vi "Facade.vi"(0 "Data In":T4, 2 "Display State In":T2, 3 "Container State":T3) -> (6 "Data Out":T4, 7 "Display State Out":T2, 8 "Action":T1)   [LabVIEW 2020, in "TTL XCtrl.xctl"]
uses:
  TTL XCtrl.xctl
  Data.vi
  TTL VIs/Control Classes/Base Class/TTLController.lvclass
  <vilib>/_xctls/Container State.ctl
  State.vi
  TTL VIs/Device Classes/Base Class/TTLControlledDevice.lvclass
  D:/Development/epl-vi-lib/Koop/KObject Class/KObject.lvclass
  <vilib>/_xctls/Action.ctl
  TTL VIs/Typedefs/TTLController XControl/TTLController.xctl
  TTL VIs/Control Classes/TTLWaterController/TTLWaterController.lvclass
  D:/Development/epl-tosca/LV Source/TTL VIs/Control Classes/Base Class/TTLController.lvclass
  TTL VIs/Control Classes/Base Class/TTLController.lvclass/TTLController.ctl
  TTL VIs/Device Classes/Base Class/TTLControlledDevice.lvclass/TTLControlledDevice.ctl
  TTL VIs/Control Classes/TCPController/TCPController.lvclass
  TTL VIs/Control Classes/Base Class/Read Name.vi
  TTL VIs/Device Classes/Base Class/Read Name.vi
  TTL VIs/Control Classes/Base Class/Write Name.vi
  <vilib>/_xctls/XControlSupport.lvlib
  epl-vi-lib/Koop/KObject Class/KObject.lvclass
panel:
  in  "TTL1":refnum<class "TTLController.lvclass">(xcontrol)
  in  "TTL2":refnum<class "TTLController.lvclass">(xcontrol)
  in  "TTL3":refnum<class "TTLController.lvclass">(xcontrol)
  in  "TTL4":refnum<class "TTLController.lvclass">(xcontrol)
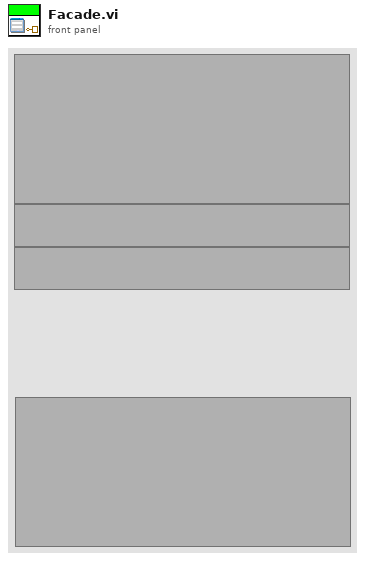
[diagram p1: front panel]
types:
  T1 = typedef "XControlSupport.lvlib/Action.ctl" = cluster{"Data Changed?":bool, "State Changed?":bool, "Action Name":string}
  T2 = typedef "TTL XCtrl.xctl/State.vi" = cluster{"Devices":refnum<class "TTLControlledDevice.lvclass">[], "action":string}
  T3 = typedef "XControlSupport.lvlib/Container State.ctl" = cluster{"Indicator?":bool, "Run Mode?":bool, " Refnum":refnum<vi>}
  T4 = typedef "TTL XCtrl.xctl/Data.vi" = refnum<class "TTLController.lvclass">[]
  T5 = enum16{"Always On", "Always Off", "Off While Running"}
  T6 = typedef "LVRectTypeDef.ctl" = cluster{"Left":i16, "Top":i16, "Right":i16, "Bottom":i16}
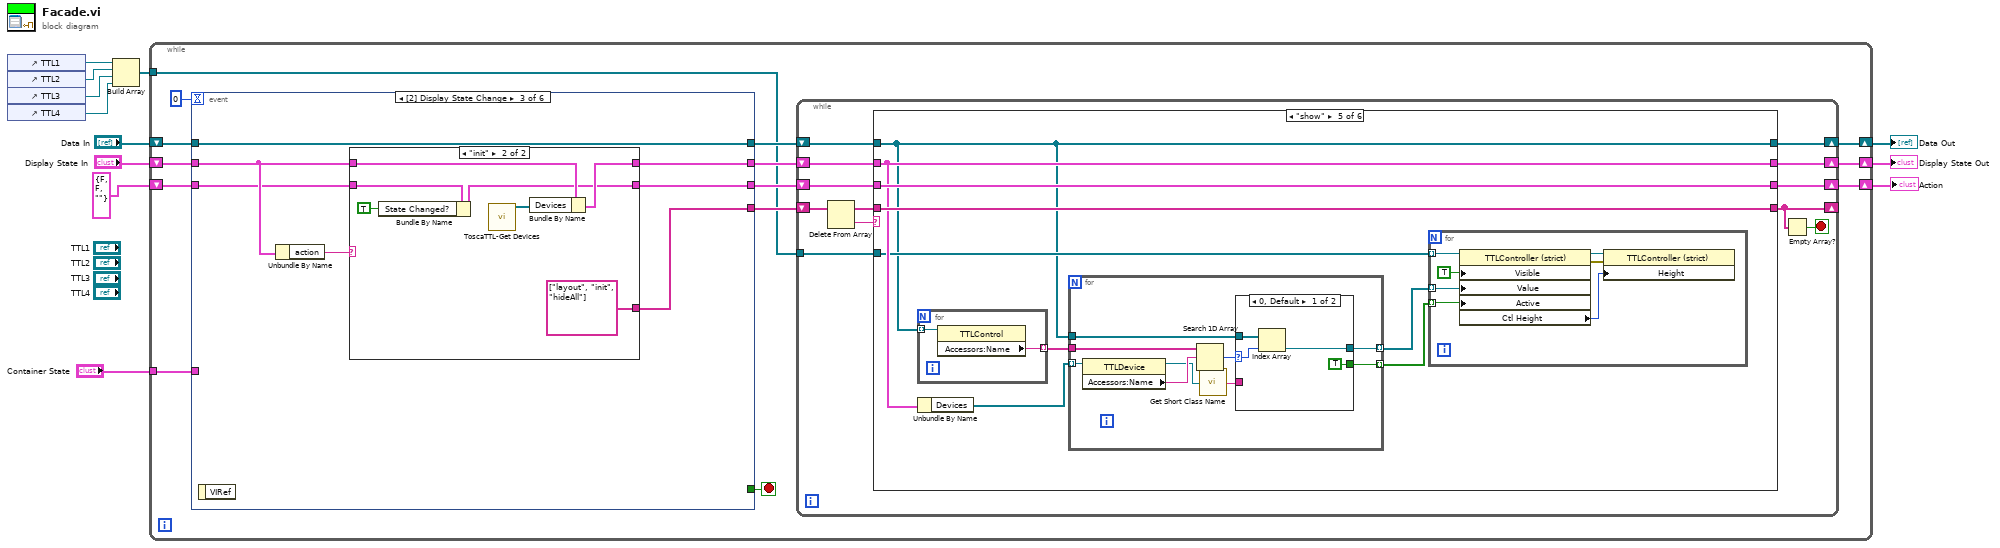
[diagram p0: block diagram]
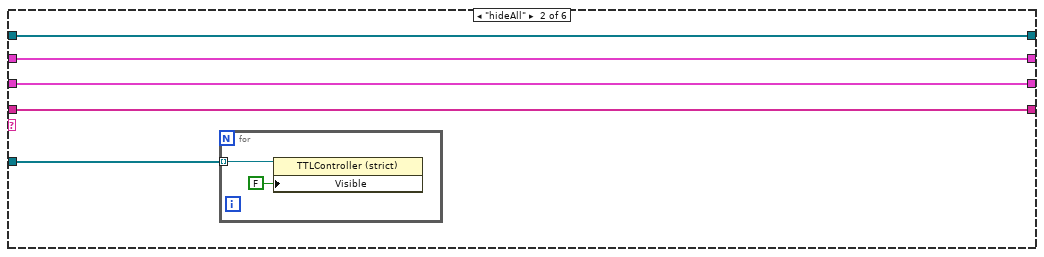
[diagram p3: hidden frame]
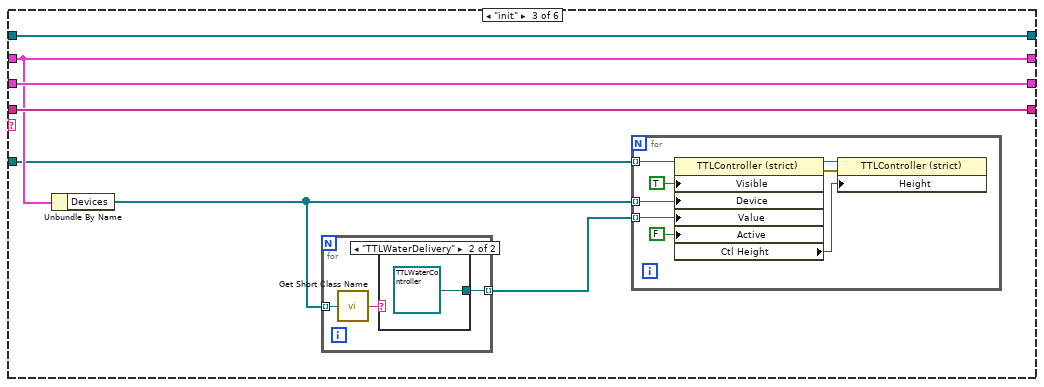
[diagram p4: hidden frame]
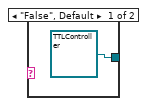
[diagram p5: hidden frame]
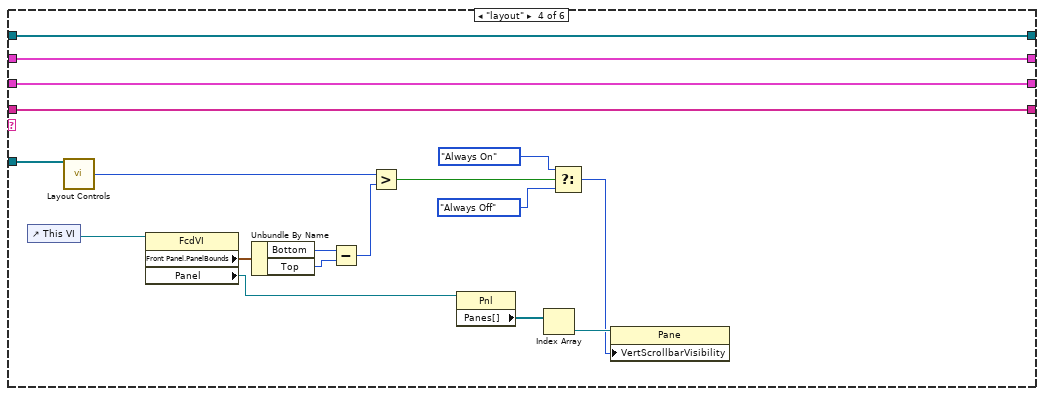
[diagram p6: hidden frame]
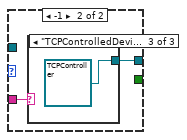
[diagram p7: hidden frame]
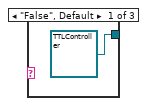
[diagram p8: hidden frame]
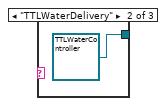
[diagram p9: hidden frame]
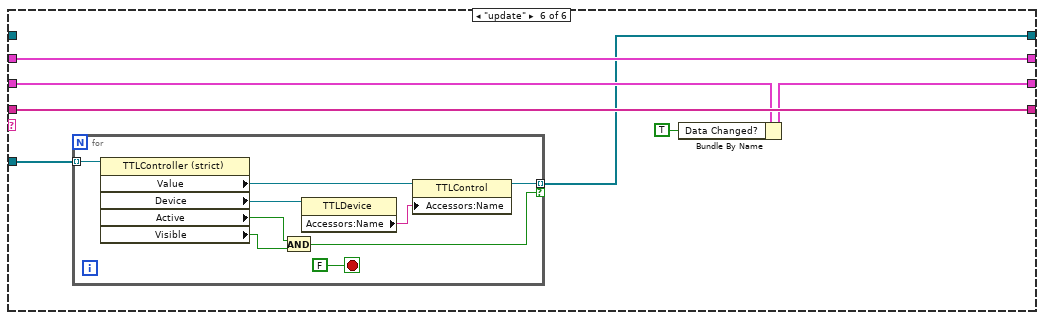
[diagram p10: hidden frame]
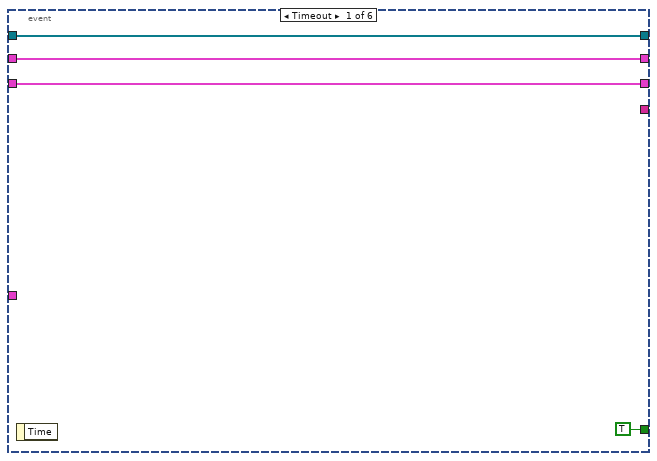
[diagram p11: hidden frame]
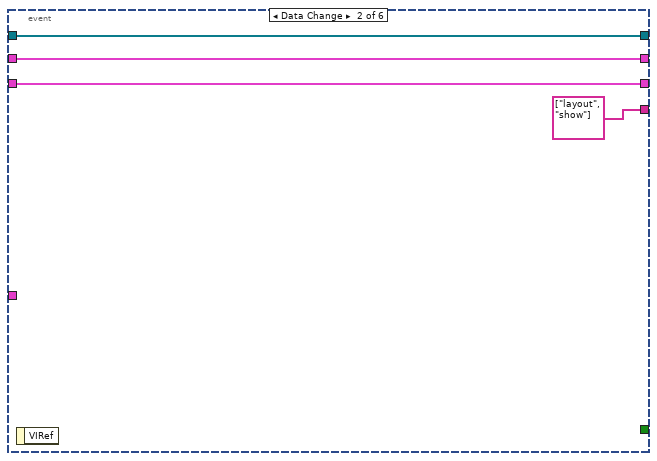
[diagram p12: hidden frame]
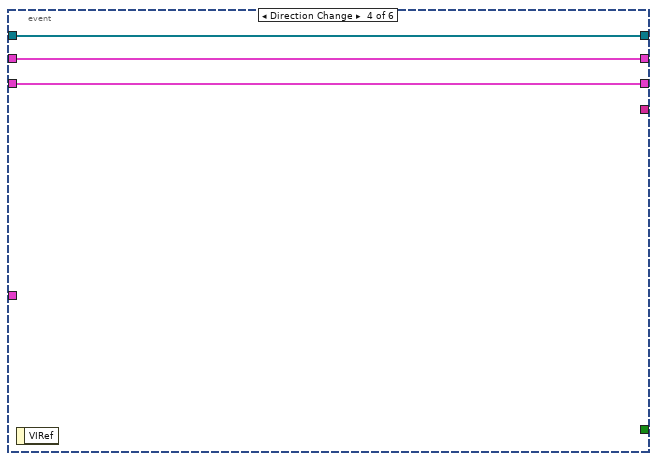
[diagram p14: hidden frame]
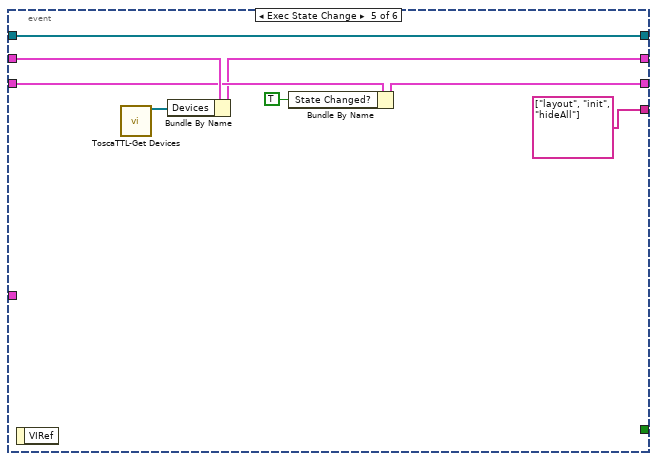
[diagram p15: hidden frame]
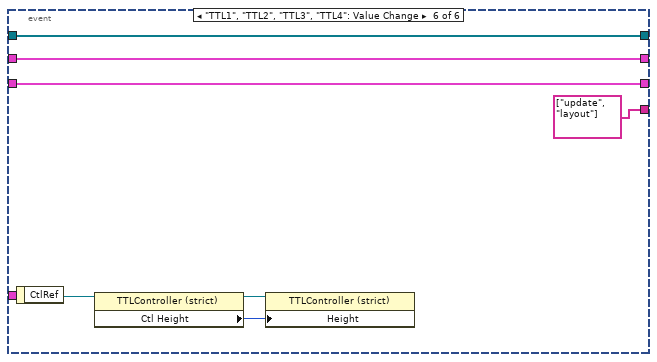
[diagram p16: hidden frame]
diagram:
  n1 = control-ref of="TTL1"() -> (w5:refnum<vi>)
  n2 = control-ref of="TTL2"() -> (w4:refnum<vi>)
  n3 = control-ref of="TTL3"() -> (w3:refnum<vi>)
  n4 = control-ref of="TTL4"() -> (w2:refnum<vi>)
  n5 = Build Array(w5, w4, w3, w2) -> (w1:refnum<vi>[])
  n6 = while {
    shift-right: [w15] -> w9
    shift-left: "Display State In" -> [w26]
    tunnel: "Container State" -> [w23]
    shift-right: [w16] -> w12
    shift-left: "Data In" -> [w22]
    shift-right: [w14] -> w7
    shift-left: T1 {"Data Changed?"=FALSE, "State Changed?"=FALSE, "Action Name"=""} ("Action") -> [w21]
    tunnel: w1 -> [w13]
    stop <- w25 stop-if-true
    n7 = event shown="[2] Display State Change" {
      selector: _ -> [_ _ _ _ _ _]
      dyn-events: _ -> [_ _ _ _ _ _]
      timeout: 0 -> [_ _ _ _ _ _]
      tunnel: w26 -> [w141 w145 w152 w166 w174 w175]
      tunnel: [w141 w145 w150 w166 w171 w175] -> w18
      tunnel: [TRUE _ _ _ _ _] -> w25
      tunnel: w23 -> [_ _ _ _ _ _]
      tunnel: w22 -> [w140 w144 w154 w165 w173 w181]
      tunnel: [w140 w144 w154 w165 w173 w181] -> w19
      tunnel: [w142 w147 w149 w164 w169 w180] -> w17
      tunnel: w21 -> [w142 w147 w151 w164 w172 w180]
      tunnel: [_ string[] ["layout", "show"] w148 _ string[] ["layout", "init", "hideAll"] string[] ["update", "layout"]] -> w20
      event Timeout {
        n8 = event-data() -> ()  [unwired: 1 in, 1 out]
      }
      event Data Change {
        n9 = event-data() -> ()  [unwired: 1 in, 1 out]
      }
      event Display State Change {
        n10 = event-data() -> ()  [unwired: 1 in, 1 out]
        n11 = Unbundle By Name(w152) -> ("action"=w153:string)
        n12 = case shown="\"init\"" w153 {
          tunnel: w152 -> [w156 w160]
          tunnel: w151 -> [w155 w158]
          tunnel: [w156 w159] -> w150
          tunnel: [w155 w157] -> w149
          tunnel: [_ string[] ["layout", "init", "hideAll"]] -> w148
          frame "", Default {
          }
          frame "init" {
            n13 = Bundle By Name(cluster=w158, "State Changed?"=TRUE) -> (w157:T1)
            n14 = call "ToscaTTL-Get Devices.vi"() -> ("Devices"=w163:refnum<class "TTLControlledDevice.lvclass">[])  [unwired: 12 in, 3 out]
            n15 = Bundle By Name(cluster=w160, "Devices"=w163) -> (w159:T2)
          }
        }
      }
      event Direction Change {
        n16 = event-data() -> ()  [unwired: 1 in, 1 out]
      }
      event Exec State Change {
        n17 = event-data() -> ()  [unwired: 1 in, 1 out]
        n18 = call "ToscaTTL-Get Devices.vi"() -> ("Devices"=w170:refnum<class "TTLControlledDevice.lvclass">[])  [unwired: 12 in, 3 out]
        n19 = Bundle By Name(cluster=w174, "Devices"=w170) -> (w171:T2)
        n20 = Bundle By Name(cluster=w172, "State Changed?"=TRUE) -> (w169:T1)
      }
      event "TTL1", "TTL2", "TTL3", "TTL4": Value Change {
        n21 = event-data() -> ("CtlRef"=w179:refnum<vi>)  [unwired: 1 in]
        n22 = property class="TTLController (strict)"(reference=w179) -> (reference out=w178:refnum<vi>, "Ctl Height"=w177:i32)  [unwired: 1 in, 1 out]
        n23 = property class="TTLController (strict)"(reference=w178, "Height"=w177) -> ()  [unwired: 1 in, 2 out]
      }
    }
    n24 = while {
      shift-right: [w35] -> _
      shift-left: w20 -> [w38]
      shift-right: [w28] -> w14
      shift-left: w17 -> [w31]
      shift-right: [w29] -> w15
      shift-left: w18 -> [w32]
      shift-right: [w30] -> w16
      shift-left: w19 -> [w33]
      tunnel: w13 -> [w27]
      stop <- w34 stop-if-true
      n25 = Delete From Array(array=w38) -> (deleted portion=w36:string, array with subset deleted=w37:string[])  [unwired: 2 in]
      n26 = case shown="\"show\"" w36 {
        tunnel: w37 -> [w42 w47 w56 w87 w96 w130]
        tunnel: [w42 w47 w56 w87 w96 w130] -> w35
        tunnel: w33 -> [w39 w46 w55 w86 w89 _]
        tunnel: w32 -> [w40 w45 w53 w85 w94 w129]
        tunnel: w31 -> [w41 w44 w54 w84 w95 w128]
        tunnel: [w39 w46 w55 w86 w89 w126] -> w30
        tunnel: [w40 w45 w53 w85 w94 w129] -> w29
        tunnel: [w41 w44 w54 w84 w95 w125] -> w28
        tunnel: w27 -> [_ w43 w52 w83 w93 w127]
        frame "", Default {
        }
        frame "hideAll" {
          n27 = for {
            tunnel: w43 -> [w48] mode=indexing
            n28 = property class="TTLController (strict)"(reference=w48, "Visible"=FALSE) -> ()  [unwired: 1 in, 2 out]
          }
        }
        frame "init" {
          n29 = Unbundle By Name(w53) -> ("Devices"=w51:refnum<class "TTLControlledDevice.lvclass">[])
          n30 = for {
            tunnel: [w67] -> w50 mode=indexing
            tunnel: w51 -> [w65] mode=indexing
            n31 = call "Get Short Class Name.vi"("KObject in"=w65) -> ("Class"=w66:string)  [unwired: 4 in]
            n32 = case shown="\"TTLWaterDelivery\"" w66 {
              tunnel: [refnum<class "TTLController.lvclass"> refnum ("Cluster In") refnum<class "TTLWaterController.lvclass"> refnum ("Cluster In")] -> w67
              frame "False", Default {
              }
              frame "TTLWaterDelivery" {
              }
            }
          }
          n33 = for {
            tunnel: w52 -> [w64] mode=indexing
            tunnel: w50 -> [w62] mode=indexing
            tunnel: w51 -> [w58] mode=indexing
            n34 = property class="TTLController (strict)"(reference=w64, "Visible"=TRUE, "Device"=w58, "Value"=w62, "Active"=FALSE) -> (reference out=w61:refnum<vi>, error out=w60:errorcluster, "Ctl Height"=w59:i32)  [unwired: 1 in]
            n35 = property class="TTLController (strict)"(reference=w61, error in=w60, "Height"=w59) -> ()  [unwired: 2 out]
          }
        }
        frame "layout" {
          n36 = control-ref of="This VI"() -> (w82:refnum<vi>)
          n37 = call "Layout Controls.vi"("Controls"=w83) -> ("Height"=w78:u32)  [unwired: 14 in]
          n38 = property class="FcdVI"(reference=w82) -> ("Front Panel.PanelBounds"=w81:T6, "Panel"=w76:refnum<vi>)  [unwired: 1 in, 2 out]
          n39 = Unbundle By Name(w81) -> ("Bottom"=w80:i16, "Top"=w79:i16)
          n40 = Subtract(x=w80, y=w79) -> (x-y=w77:i16)
          n41 = Greater?(x=w78, y=w77) -> (0:w73:bool)
          n42 = property class="Pnl"(reference=w76) -> ("Panes[]"=w75:refnum<vi>[])  [unwired: 1 in, 2 out]
          n43 = Index Array(array=w75) -> (element=w74:refnum<vi>)  [unwired: 1 in]
          n44 = Select(t=T5."Always On" ("Vertical Scrollbar Visibility"), s=w73, f=T5."Always Off") -> (s? t:f=w71:T5)
          n45 = property class="Pane"(reference=w74, "VertScrollbarVisibility"=w71) -> ()  [unwired: 1 in, 2 out]
        }
        frame "show" {
          n46 = for {
            tunnel: w89 -> [w116] mode=indexing
            tunnel: [w115] -> w91 mode=indexing
            n47 = property class="TTLControl"(reference=w116) -> ("Accessors:Name"=w115:string)  [unwired: 1 in, 2 out]
          }
          n48 = Unbundle By Name(w94) -> ("Devices"=w92:refnum<class "TTLControlledDevice.lvclass">[])
          n49 = for {
            tunnel: w92 -> [w105] mode=indexing
            tunnel: w91 -> [w104]
            tunnel: w89 -> [w102]
            tunnel: [w101] -> w90 mode=indexing
            tunnel: [w97] -> w88 mode=indexing
            n50 = property class="TTLDevice"(reference=w105) -> (reference out=w99:refnum<class "TTLControlledDevice.lvclass">, "Accessors:Name"=w100:string)  [unwired: 1 in, 1 out]
            n51 = Search 1D Array(1D array=w104, element=w100) -> (index of element=w103:i32)  [unwired: 1 in]
            n52 = call "Get Short Class Name.vi"("KObject in"=w99) -> ("Class"=w98:string)  [unwired: 4 in]
            n53 = case shown="0, Default" w103 {
              selector: w103 -> [w108 _]
              tunnel: w102 -> [w109 _]
              tunnel: [w107 w110] -> w101
              tunnel: w98 -> [_ w111]
              tunnel: [TRUE _] -> w97
              frame 0, Default {
                n54 = Index Array(array=w109, index=w108) -> (element=w107:refnum<class "TTLController.lvclass">)
              }
              frame -1 {
                n55 = case shown="\"TCPControlledDevice\"" w111 {
                  tunnel: [refnum<class "TTLController.lvclass"> refnum ("Cluster In") refnum<class "TTLWaterController.lvclass"> refnum ("Cluster In") refnum<class "TCPController.lvclass"> refnum ("TCPController")] -> w110
                  frame "False", Default {
                  }
                  frame "TTLWaterDelivery" {
                  }
                  frame "TCPControlledDevice" {
                  }
                }
              }
            }
          }
          n56 = for {
            tunnel: w93 -> [w123] mode=indexing
            tunnel: w90 -> [w118] mode=indexing
            tunnel: w88 -> [w117] mode=indexing
            n57 = property class="TTLController (strict)"(reference=w123, "Visible"=TRUE, "Value"=w118, "Active"=w117) -> (reference out=w121:refnum<vi>, error out=w120:errorcluster, "Ctl Height"=w119:i32)  [unwired: 1 in]
            n58 = property class="TTLController (strict)"(reference=w121, error in=w120, "Height"=w119) -> ()  [unwired: 2 out]
          }
        }
        frame "update" {
          n59 = for {
            tunnel: w127 -> [w139] mode=indexing
            tunnel: [w133] -> w126 mode=indexing if=w137
            stop <- FALSE stop-if-true
            n60 = property class="TTLController (strict)"(reference=w139) -> ("Value"=w134:refnum<class "TTLController.lvclass">, "Device"=w132:refnum<class "TTLControlledDevice.lvclass">, "Active"=w136:bool, "Visible"=w138:bool)  [unwired: 1 in, 2 out]
            n61 = And(x=w136, y=w138) -> (x .and. y?=w137:bool)
            n62 = property class="TTLDevice"(reference=w132) -> ("Accessors:Name"=w131:string)  [unwired: 1 in, 2 out]
            n63 = property class="TTLControl"(reference=w134, "Accessors:Name"=w131) -> (reference out=w133:refnum<class "TTLController.lvclass">)  [unwired: 1 in, 1 out]
          }
          n64 = Bundle By Name(cluster=w128, "Data Changed?"=TRUE) -> (w125:T1)
        }
      }
      n65 = Empty Array?(array=w35) -> (empty?=w34:bool)
    }
  }
  "Display State Out" <- w9
  "Data Out" <- w12
  "Action" <- w7
